vi "Create All Message Queues.vi"(8 "error in (no error)":T1 caption="entrée d'erreur (pas d'erreur)", 11 "Événement utilisateur - Arrêt":refnum<user-event>) -> (0 "error out":T1 caption="sortie d'erreur", 3 "Files d'attente de messages en sortie":T2)   [LabVIEW 2020, in "Message Queue.lvlib"]
doc: "Ce VI crée et initialise toutes les files d'attente de messages de l'application. Si votre application requiert plusieurs files d'attente de messages, cliquez sur la constante \"Message Queues\" ci-dessus avec le bouton droit et sélectionnez Ouvrir la déf. de type. Ajoutez les nouvelles files d'attente de messages à la définition de type puis initialisez-les dans ce VI."
uses:
  Message Queue.lvlib
  All Message Queues.ctl
  Message Cluster.ctl
  Enqueue Message (Single).vi
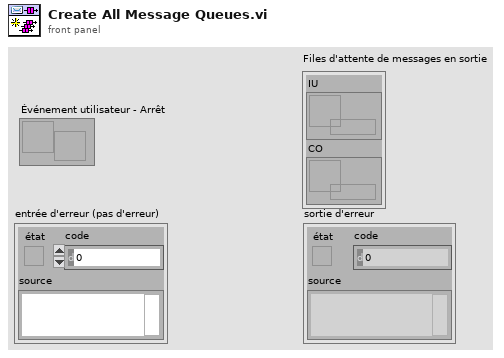
[diagram p1: front panel]
types:
  T1 = cluster{"état":bool, "code":i32, "source":string}
  T2 = typedef "Message Queue.lvlib/All Message Queues.ctl" = cluster{"IU":refnum<queue>, "CO":refnum<queue>}
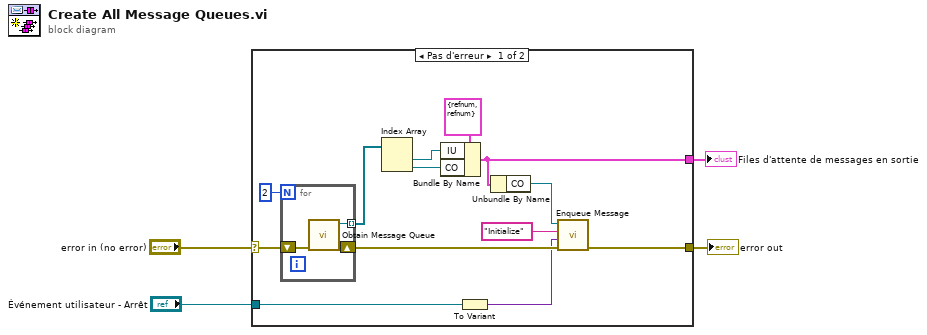
[diagram p0: block diagram]
diagram:
  n1 = case shown="Pas d'erreur" "error in (no error)" {
    selector: "error in (no error)" -> [w15 w21]
    tunnel: [w17 w21] -> w4
    tunnel: [w6 _] -> w3
    tunnel: "Événement utilisateur - Arrêt" -> [w8 _]
    frame No Error {
      n2 = for {
        N: 2 -> [_]
        tunnel: [w18] -> w11 mode=indexing
        shift-right: [w19] -> w14
        shift-left: w15 -> [w20]
        n3 = call "Obtain Message Queue.vi"("error in (no error)"=w20) -> ("error out"=w19:T1, "File d'attente de messages"=w18:refnum<queue>)  [unwired: 9 in]
      }
      n4 = Index Array(array=w11) -> (element #1=w10:refnum<queue>, element #2=w9:refnum<queue>)  [unwired: 2 in]
      n5 = Bundle By Name(cluster=T2 {"IU"=refnum, "CO"=refnum} ("Files d'attente de messages"), "IU"=w10, "CO"=w9) -> (w6:T2)
      n6 = To Variant(anything=w8) -> (Variant=w7:variant)
      n7 = Unbundle By Name(w6) -> ("CO"=w5:refnum<queue>)
      n8 = call-poly "Enqueue Message.vi"("error in (no error)"=w14, "Données de message"=w7, "Message"="Initialize", "File d'attente de messages"=w5) -> ("error out"=w17:T1)  [unwired: 6 in, 1 out]
    }
    frame Error {
    }
  }
  "Files d'attente de messages en sortie" <- w3
  "error out" <- w4
